vi "Test Pause Refreshing Trigger Broadcast.vi"(8 "error in (no error)":errorcluster, 11 "Test Case In":refnum<class "Debugger Test.lvclass">) -> (0 "error out":errorcluster, 3 "Test Case Out":refnum<class "Debugger Test.lvclass">)   [LabVIEW 2020, in "Debugger Test.lvclass"]
uses:
  Debugger Test.lvclass
  C:/Program Files (x86)/National Instruments/LabVIEW 2020/vi.lib/Astemes/LUnit/Test Case.lvclass
  source/Debugger/Debugger.lvclass
  C:/Git/astemes-triarc-debugger/source/Process/Debug Process.lvclass
  source/Process/Debug Process.lvclass/Debug Process.ctl
  <vilib>/Astemes/LUnit/Test Case.lvclass/Test Case.ctl
  01074fa8-ee8a-411d-bc8b-fc92c4f90959.vi
  source/Process/Public/Lifecycle/Get Lifecycle State.vi
  <vilib>/Astemes/Triarc Framework/Broadcast Event Helpers/Execution timer.vi
  source/Process/Private/SubVIs/Wait for finish.vi
  source/Process/Protected/Messaging/Enqueue Message.vi
  source/Process/Private/SubVIs/Set Lifecycle State.vi
  <vilib>/Astemes/LUnit/Palette/Pass.vi
  <vilib>/Astemes/LUnit/Palette/Fail.vi
  <vilib>/Astemes/LUnit/Compare Variants.vi
  <vilib>/Astemes/LUnit/Describe Comparison.vi
  <vilib>/Astemes/LUnit/Set Assertion Type.vi
  <vilib>/Utility/error.llb/Clear Errors.vi
  <vilib>/Astemes/LUnit/Add test result.vi
  <vilib>/Astemes/LUnit/Variant to string.vi
  <vilib>/Astemes/LUnit/LUnit Record Assertion Result.vi
  <vilib>/Astemes/LUnit/LUnit Aggregate Assertion Results.vi
  <vilib>/Astemes/LUnit/Method Result/LUnit Merge Status.vi
  <vilib>/Astemes/LUnit/LUnit Concatenate result strings.vi
  <vilib>/Utility/error.llb/Error Cluster From Error Code.vi
  <vilib>/Astemes/Triarc Framework/Broadcast Event Helpers/Dequeue Broadcast Message.vi
  <vilib>/Utility/Data Type/Get Type Information.vi
  <vilib>/Utility/LVClass/Get LV Class Name.vi
  source/Process/Debug Process.lvclass
  Debugger Test.lvclass/Debugger Test.ctl
  <vilib>/Astemes/Triarc Framework/Broadcast Event Helpers/Broadcast Event Helpers.lvlib
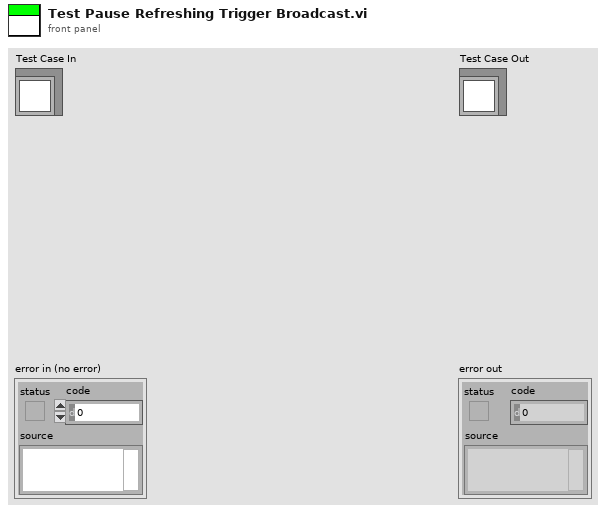
[diagram p1: front panel]
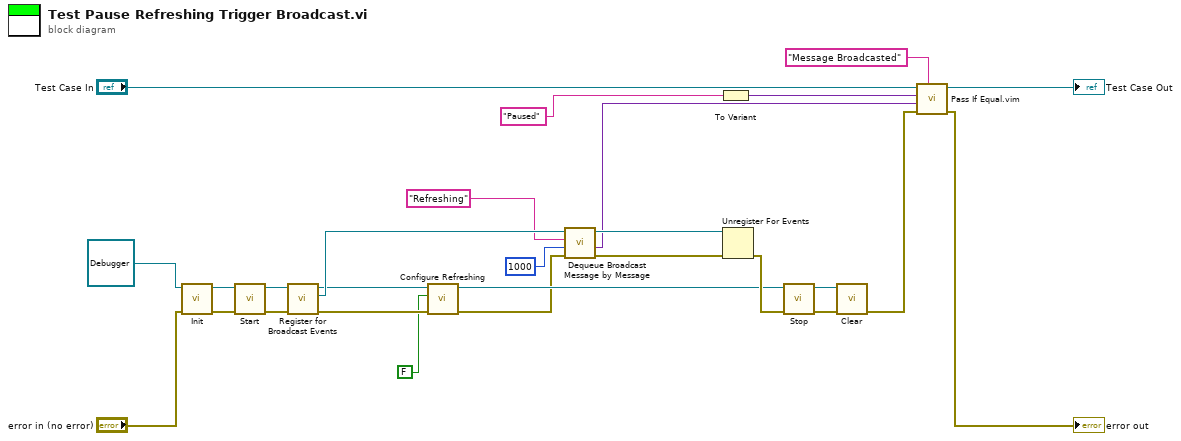
[diagram p0: block diagram]
diagram:
  n1 = call-dynamic "Init.vi"("error in (no error)"="error in (no error)", "Process In"=refnum<class "Debugger.lvclass"> refnum ("Debug Data Event In 2")) -> ("error out"=w23:errorcluster, "Process Out"=w24:refnum<class "Debugger.lvclass">)  [unwired: 8 in]
  n2 = call "Start.vi"("error in (no error)"=w23, "Process In"=w24) -> ("error out"=w21:errorcluster, "Process Out"=w22:refnum<class "Debugger.lvclass">)  [unwired: 7 in, 1 out]
  n3 = call "Register for Broadcast Events.vi"("error in (no error)"=w21, "Process In"=w22) -> ("error out"=w13:errorcluster, "Event Registration Refnum Out"=w14:refnum<event-registration>, "Process Out"=w12:refnum<class "Debugger.lvclass">)  [unwired: 7 in]
  n4 = call "Configure Refreshing.vi"("error in (no error)"=w13, "Refresh?"=FALSE ("Show Send?"), "Debugger In"=w12) -> ("error out"=w4:errorcluster, "Debugger Out"=w5:refnum<class "Debugger.lvclass">)  [unwired: 7 in]
  n5 = call <vilib>:"Dequeue Broadcast Message by Message.vi"("error in (no error)"=w4, "Timeout (-1)"=1000, "Message"="Refreshing", "Event Registration Refnum"=w14) -> ("error out"=w6:errorcluster, "Message Data"=w3:variant, "Event Registration Refnum Out"=w9:refnum<event-registration>)  [unwired: 3 in, 2 out]
  n6 = To Variant(anything="Paused" ("Message")) -> (Variant=w1:variant)
  n7 = Unregister For Events(event registration refnum=w9, error in=w6) -> (error out=w11:errorcluster)
  n8 = call "Stop.vi"("error in (no error)"=w11, "Process In"=w5) -> ("error out"=w19:errorcluster, "Process Out"=w20:refnum<class "Debugger.lvclass">)  [unwired: 7 in, 1 out]
  n9 = call-dynamic "Clear.vi"("error in (no error)"=w19, "Process In"=w20) -> ("error out"=w16:errorcluster)  [unwired: 9 in]
  n10 = call "Pass If Equal.vim"("Description"="Message Broadcasted", "error in (no error)"=w16, "Actual"=w3, "Expected"=w1, "LUnit Test Case In"="Test Case In") -> ("error out"=→"error out":errorcluster, "LUnit Test Case Out"=→"Test Case Out":refnum<class "Debugger Test.lvclass">)  [unwired: 5 in]
